vi "LSCI 370 Config Control Parameters.vi"(0 "VISA session":refnum<visa-resource-name>, 1 "Manual Output (0.000)":dbl min=0.0 max=100.0 step=0.001 format="%.3f", 2 "Heater Range (0: Off)":u16(ring) items=["Off", "31.6 uA", "100 uA", "316 uA", "1.00 mA", "3.16 mA", "10.0 mA", "31.6 mA", "100 mA"], 7 "Gain (P) (10.000)":dbl=10.0 min=0.001 max=1000.0 step=0.001 format="%.3f", 9 "Reset (I) (20)":dbl=20.0 min=0.0 max=10000.0 step=1.0, 11 "error in (no error)":errorcluster, 12 "Rate (D) (0)":dbl min=0.0 max=2500.0 step=1.0) -> (4 "dup VISA session":refnum<visa-resource-name>, 15 "error out":errorcluster)   [LabVIEW 2016]
doc: "This VI Configures the 370 Control Parameters, functions configured are PID, Heater Range, and Manual Output."
panel:
  # "%"
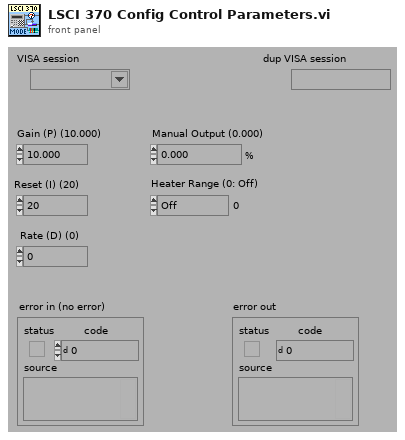
[diagram p1: front panel]
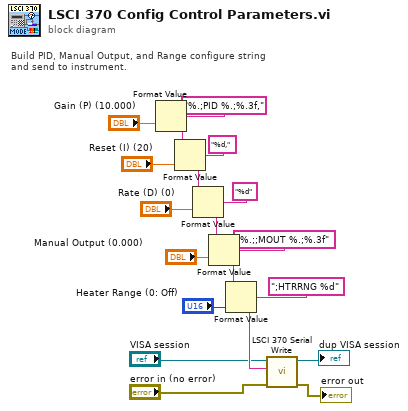
[diagram p0: block diagram]
diagram:
  # "Build PID, Manual Output, and Range configure string\nand send to instrument."
  n1 = Format Value(format string="%.;PID %.;%.3f,", value (0)="Gain (P) (10.000)") -> (output string=w15:string)  [unwired: 1 in]
  n2 = Format Value(string ("")=w15, format string="%d,", value (0)="Reset (I) (20)") -> (output string=w14:string)
  n3 = Format Value(string ("")=w14, format string="%d", value (0)="Rate (D) (0)") -> (output string=w3:string)
  n4 = Format Value(string ("")=w3, format string="%.;;MOUT %.;%.3f", value (0)="Manual Output (0.000)") -> (output string=w9:string)
  n5 = Format Value(string ("")=w9, format string=";HTRRNG %d", value (0)="Heater Range (0: Off)") -> (output string=w8:string)
  n6 = call "LSCI 370 Serial Write.vi"("error in (no error)"="error in (no error)", "Write Buffer (\"\")"=w8, "VISA session"="VISA session") -> ("error out"=→"error out":errorcluster, "dup VISA session"=→"dup VISA session":refnum<visa-resource-name>)  [unwired: 6 in, 1 out]
